vi "Write_Component_Power.vi"(0 "AccelNET.lvlib:TCP.lvclass":refnum<class "TCP.lvclass">, 2 "Component Power":T1, 3 "error in (no error)":errorcluster) -> (10 "Error Out":errorcluster)   [LabVIEW 2012, in "AccelNET.lvlib" / "TCP.lvclass"]
uses:
  TCP.lvclass
  Component_Power_Control.ctl
  Useful_SubVIs.lvlib
  Useful_Controls.lvlib
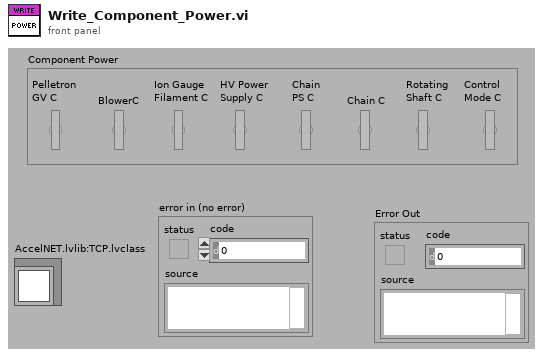
[diagram p1: front panel]
types:
  T1 = typedef "AccelNET.lvlib/Useful_Controls.lvlib/Component_Power_Control.ctl" = cluster{"Pelletron\nGV C":bool, "BlowerC":bool, "Chain C":bool, "Rotating\nShaft C":bool, "HV Power\nSupply C":bool, "Ion Gauge\nFilament C":bool, "Control\nMode C":bool, "Chain\nPS C":bool}
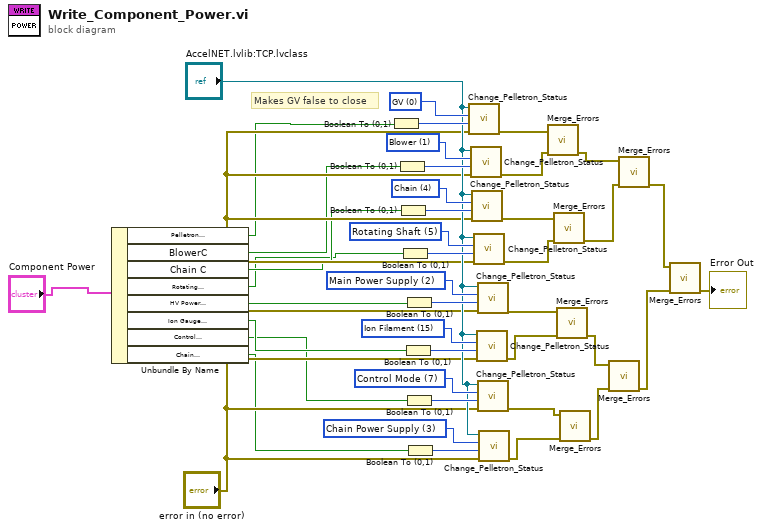
[diagram p0: block diagram]
diagram:
  w28 = u16 3 items=["GV", "Blower", "Main Power Supply", "Chain Power Supply", "Chain", "Rotating Shaft", "Power Supply Voltage", "Control Mode", "Control Mode Reference", "Chain Bypass", "Rotating Shaft Bypass", "Spark Counter", "Spark Limit", "Threshold", "Spark Counter Reset", "Ion Filament"] ("Write Selector")
  w30 = u16 7 items=["GV", "Blower", "Main Power Supply", "Chain Power Supply", "Chain", "Rotating Shaft", "Power Supply Voltage", "Control Mode", "Control Mode Reference", "Chain Bypass", "Rotating Shaft Bypass", "Spark Counter", "Spark Limit", "Threshold", "Spark Counter Reset", "Ion Filament"] ("Write Selector")
  w32 = u16 15 items=["GV", "Blower", "Main Power Supply", "Chain Power Supply", "Chain", "Rotating Shaft", "Power Supply Voltage", "Control Mode", "Control Mode Reference", "Chain Bypass", "Rotating Shaft Bypass", "Spark Counter", "Spark Limit", "Threshold", "Spark Counter Reset", "Ion Filament"] ("Write Selector")
  w34 = u16 2 items=["GV", "Blower", "Main Power Supply", "Chain Power Supply", "Chain", "Rotating Shaft", "Power Supply Voltage", "Control Mode", "Control Mode Reference", "Chain Bypass", "Rotating Shaft Bypass", "Spark Counter", "Spark Limit", "Threshold", "Spark Counter Reset", "Ion Filament"] ("Write Selector")
  w36 = u16 5 items=["GV", "Blower", "Main Power Supply", "Chain Power Supply", "Chain", "Rotating Shaft", "Power Supply Voltage", "Control Mode", "Control Mode Reference", "Chain Bypass", "Rotating Shaft Bypass", "Spark Counter", "Spark Limit", "Threshold", "Spark Counter Reset", "Ion Filament"] ("Write Selector")
  w40 = u16 4 items=["GV", "Blower", "Main Power Supply", "Chain Power Supply", "Chain", "Rotating Shaft", "Power Supply Voltage", "Control Mode", "Control Mode Reference", "Chain Bypass", "Rotating Shaft Bypass", "Spark Counter", "Spark Limit", "Threshold", "Spark Counter Reset", "Ion Filament"] ("Write Selector")
  w41 = u16 1 items=["GV", "Blower", "Main Power Supply", "Chain Power Supply", "Chain", "Rotating Shaft", "Power Supply Voltage", "Control Mode", "Control Mode Reference", "Chain Bypass", "Rotating Shaft Bypass", "Spark Counter", "Spark Limit", "Threshold", "Spark Counter Reset", "Ion Filament"] ("Write Selector")
  w42 = u16 0 items=["GV", "Blower", "Main Power Supply", "Chain Power Supply", "Chain", "Rotating Shaft", "Power Supply Voltage", "Control Mode", "Control Mode Reference", "Chain Bypass", "Rotating Shaft Bypass", "Spark Counter", "Spark Limit", "Threshold", "Spark Counter Reset", "Ion Filament"] ("Write Selector")
  # "Makes GV false to close"
  n1 = Unbundle By Name("Component Power") -> ("Pelletron\nGV C"=w1:bool, "BlowerC"=w8:bool, "Chain C"=w7:bool, "Rotating\nShaft C"=w6:bool, "HV Power\nSupply C"=w5:bool, "Ion Gauge\nFilament C"=w4:bool, "Control\nMode C"=w3:bool, "Chain\nPS C"=w2:bool)
  n2 = Boolean To (0,1)(Boolean=w1) -> (0, 1=w39:i16)
  n3 = Boolean To (0,1)(Boolean=w8) -> (0, 1=w38:i16)
  n4 = Boolean To (0,1)(Boolean=w7) -> (0, 1=w37:i16)
  n5 = Boolean To (0,1)(Boolean=w6) -> (0, 1=w35:i16)
  n6 = Boolean To (0,1)(Boolean=w4) -> (0, 1=w31:i16)
  n7 = Boolean To (0,1)(Boolean=w5) -> (0, 1=w33:i16)
  n8 = Boolean To (0,1)(Boolean=w3) -> (0, 1=w29:i16)
  n9 = Boolean To (0,1)(Boolean=w2) -> (0, 1=w27:i16)
  n10 = call "Change_Pelletron_Status.vi"("error in (no error)"="error in (no error)", "Write Value"=w39, "Write Selector"=w42, "AccelNET.lvlib:TCP.lvclass"="AccelNET.lvlib:TCP.lvclass") -> ("error out"=w17:errorcluster)  [unwired: 7 in]
  n11 = call "Change_Pelletron_Status.vi"("error in (no error)"="error in (no error)", "Write Value"=w38, "Write Selector"=w41, "AccelNET.lvlib:TCP.lvclass"="AccelNET.lvlib:TCP.lvclass") -> ("error out"=w18:errorcluster)  [unwired: 7 in]
  n12 = call "Change_Pelletron_Status.vi"("error in (no error)"="error in (no error)", "Write Value"=w37, "Write Selector"=w40, "AccelNET.lvlib:TCP.lvclass"="AccelNET.lvlib:TCP.lvclass") -> ("error out"=w19:errorcluster)  [unwired: 7 in]
  n13 = call "Change_Pelletron_Status.vi"("error in (no error)"="error in (no error)", "Write Value"=w35, "Write Selector"=w36, "AccelNET.lvlib:TCP.lvclass"="AccelNET.lvlib:TCP.lvclass") -> ("error out"=w20:errorcluster)  [unwired: 7 in]
  n14 = call "Change_Pelletron_Status.vi"("error in (no error)"="error in (no error)", "Write Value"=w31, "Write Selector"=w32, "AccelNET.lvlib:TCP.lvclass"="AccelNET.lvlib:TCP.lvclass") -> ("error out"=w22:errorcluster)  [unwired: 7 in]
  n15 = call "Change_Pelletron_Status.vi"("error in (no error)"="error in (no error)", "Write Value"=w33, "Write Selector"=w34, "AccelNET.lvlib:TCP.lvclass"="AccelNET.lvlib:TCP.lvclass") -> ("error out"=w21:errorcluster)  [unwired: 7 in]
  n16 = call "Change_Pelletron_Status.vi"("error in (no error)"="error in (no error)", "Write Value"=w29, "Write Selector"=w30, "AccelNET.lvlib:TCP.lvclass"="AccelNET.lvlib:TCP.lvclass") -> ("error out"=w23:errorcluster)  [unwired: 7 in]
  n17 = call "Change_Pelletron_Status.vi"("error in (no error)"="error in (no error)", "Write Value"=w27, "Write Selector"=w28, "AccelNET.lvlib:TCP.lvclass"="AccelNET.lvlib:TCP.lvclass") -> ("error out"=w24:errorcluster)  [unwired: 7 in]
  n18 = call "Merge_Errors.vi"("Error 2"=w18, "Error 1"=w17) -> ("Error Out"=w16:errorcluster)  [unwired: 9 in]
  n19 = call "Merge_Errors.vi"("Error 2"=w20, "Error 1"=w19) -> ("Error Out"=w15:errorcluster)  [unwired: 9 in]
  n20 = call "Merge_Errors.vi"("Error 2"=w22, "Error 1"=w21) -> ("Error Out"=w14:errorcluster)  [unwired: 9 in]
  n21 = call "Merge_Errors.vi"("Error 2"=w24, "Error 1"=w23) -> ("Error Out"=w13:errorcluster)  [unwired: 9 in]
  n22 = call "Merge_Errors.vi"("Error 2"=w13, "Error 1"=w14) -> ("Error Out"=w12:errorcluster)  [unwired: 9 in]
  n23 = call "Merge_Errors.vi"("Error 2"=w15, "Error 1"=w16) -> ("Error Out"=w11:errorcluster)  [unwired: 9 in]
  n24 = call "Merge_Errors.vi"("Error 2"=w12, "Error 1"=w11) -> ("Error Out"=→"Error Out":errorcluster)  [unwired: 9 in]
